vi "Chamber Edit Steptype.vi"(8 "error in":errorcluster, 10 "Chamber data in":T1, 11 "Sequence Context In":refnum<k7>) -> (0 "error out":errorcluster, 2 "Chamber data out":T1, 3 "Report Text":string)   [LabVIEW 2023, in "LTT_TeststandSteptypes.lvlib"]
uses:
  LTT_TeststandSteptypes.lvlib
  Control/Chamber Step Option.ctl
  Control/Chamber Step Status.ctl
  <vilib>/addons/TestStand/_TSUtility.llb/TestStand - Start Modal Dialog (Sequence Context).vi
  <vilib>/addons/TestStand/_TSUtility.llb/TestStand - End Modal Dialog (Sequence Context).vi
panel:
  in  "Chamber Command":T2
  in  "Close":bool
  in  "OK":bool
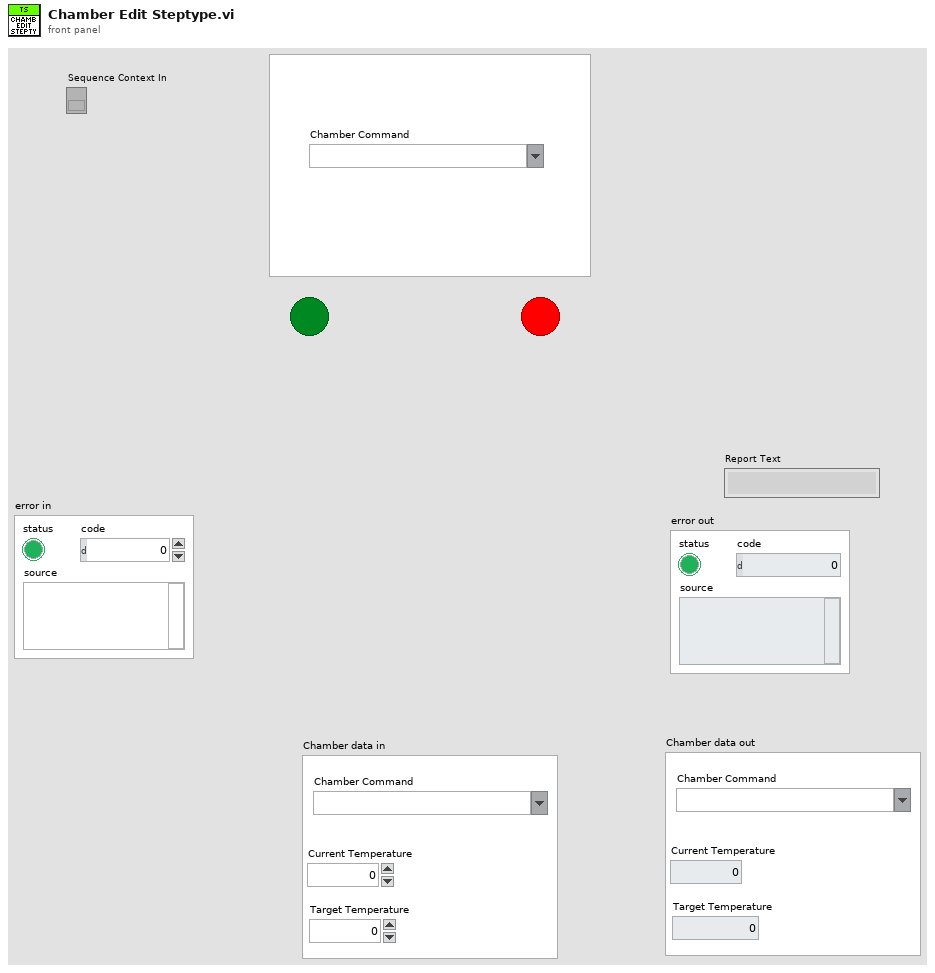
[diagram p1: front panel]
types:
  T1 = typedef "LTT_TeststandSteptypes.lvlib/Chamber Step Status.ctl" = cluster{"Current Temperature":dbl, "Target Temperature":dbl, "Chamber Command":T2}
  T2 = typedef "LTT_TeststandSteptypes.lvlib/Chamber Step Option.ctl" = string
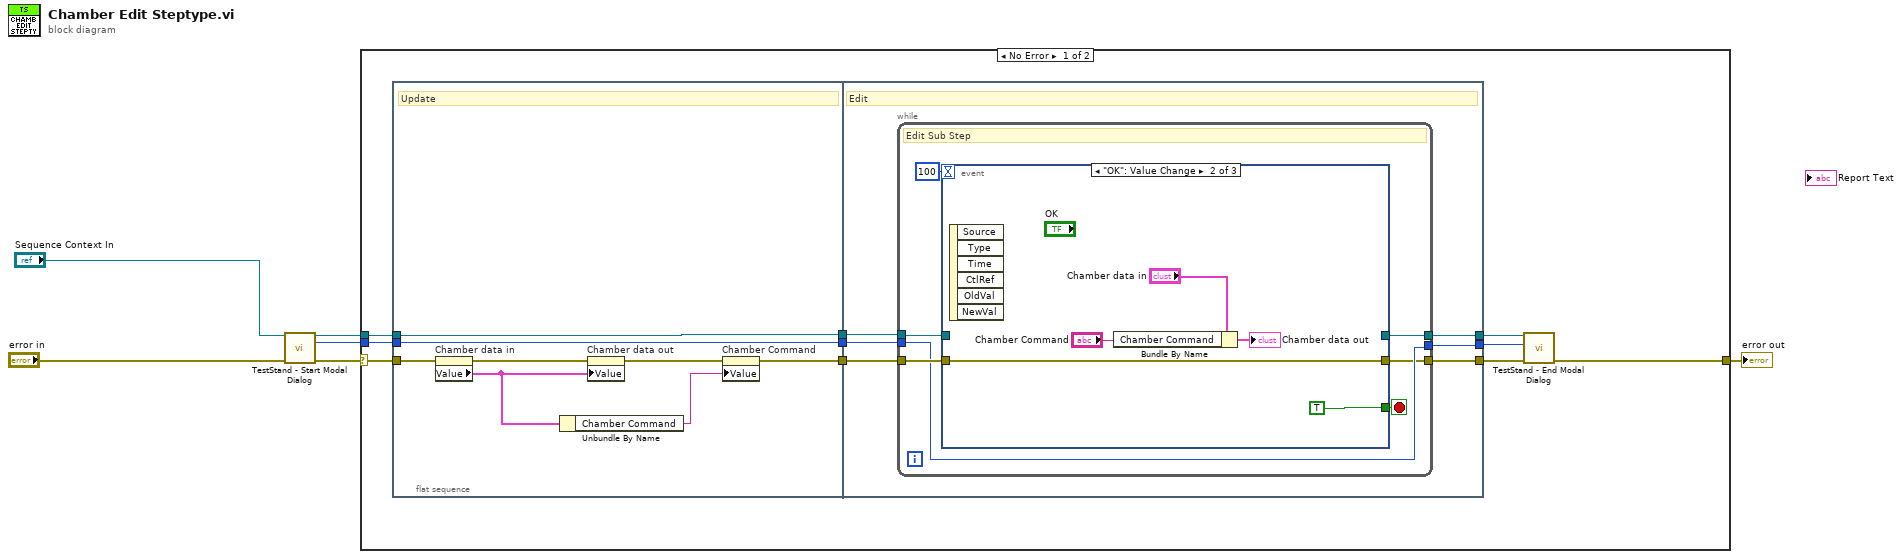
[diagram p0: block diagram]
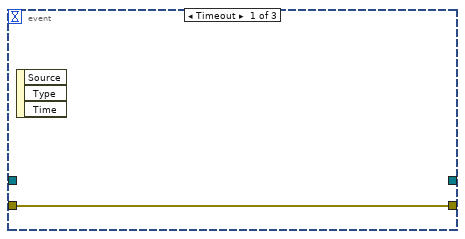
[diagram p2: hidden frame]
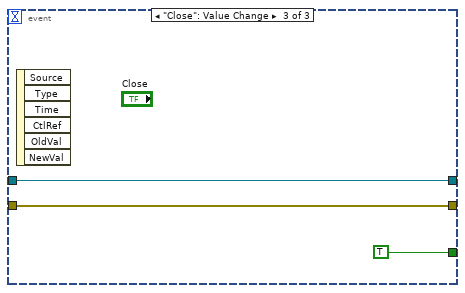
[diagram p3: hidden frame]
diagram:
  n1 = call-poly <vilib>:"TestStand - Start Modal Dialog.vi"("Sequence Context In"="Sequence Context In", "error in (no error)"="error in") -> ("Sequence Context Out"=w4:refnum<k7>, "Modal ID"=w3:i32, "error out"=w5:errorcluster)  [unwired: 9 in, 2 out]
  n2 = case shown="No Error" w5 {
    selector: w5 -> [w13 w47]
    tunnel: w4 -> [w11 _]
    tunnel: w3 -> [w10 _]
    tunnel: [w7 w47] -> w2
    frame No Error {
      n3 = flat-sequence {
        tunnel: w13 -> [w22]
        tunnel: [w18] -> w16
        tunnel: w11 -> [w24]
        tunnel: w10 -> [w23]
        tunnel: [w24] -> w15
        tunnel: [w23] -> w14
        tunnel: w16 -> [w28]
        tunnel: [w26] -> w12
        tunnel: w15 -> [w30]
        tunnel: w14 -> [w29]
        tunnel: [w27] -> w9
        tunnel: [w25] -> w8
        frame #0 {
          # "Update"
          n4 = property on="Chamber data in" class="Clust (strict)"(error in=w22) -> (error out=w21:errorcluster, "Value"=w20:T1)  [unwired: 1 in, 1 out]
          n5 = Unbundle By Name(w20) -> ("Chamber Command"=w17:T2)
          n6 = property on="Chamber data out" class="Clust (strict)"(error in=w21, "Value"=w20) -> (error out=w19:errorcluster)  [unwired: 1 in, 1 out]
          n7 = property on="Chamber Command" class="CmbBox (strict)"(error in=w19, "Value"=w17) -> (error out=w18:errorcluster)  [unwired: 1 in, 1 out]
        }
        frame #1 {
          # "Edit"
          n8 = while {
            tunnel: w30 -> [w35]
            tunnel: w29 -> [w32]
            tunnel: w28 -> [w33]
            tunnel: [w34] -> w25
            tunnel: [w32] -> w27
            tunnel: [w31] -> w26
            stop <- w36 stop-if-true
            # "Edit Sub Step"
            n9 = event shown="[1] \"OK\": Value Change" {
              selector: _ -> [_ _ _]
              dyn-events: _ -> [_ _ _]
              timeout: 100 -> [_ _ _]
              tunnel: [_ TRUE TRUE] -> w36
              tunnel: [_ _ w45] -> w34
              tunnel: w35 -> [_ _ w45]
              tunnel: w33 -> [w38 w42 w44]
              tunnel: [w38 w42 w44] -> w31
              event Timeout {
                n10 = event-data() -> ()  [unwired: 1 in, 3 out]
              }
              event "OK": Value Change {
                n11 = event-data() -> ()  [unwired: 1 in, 6 out]
                n12 = Bundle By Name(cluster="Chamber data in", "Chamber Command"="Chamber Command") -> (→"Chamber data out":T1)
              }
              event "Close": Value Change {
                n13 = event-data() -> ()  [unwired: 1 in, 6 out]
              }
            }
          }
        }
      }
      n14 = call-poly <vilib>:"TestStand - End Modal Dialog.vi"("Sequence Context In"=w8, "Modal ID"=w9, "error in (no error)"=w12) -> ("error out"=w7:errorcluster)  [unwired: 12 in]
    }
    frame Error {
    }
  }
  "error out" <- w2
